vi "Set Relay State.vi"(8 "error in (no error)":errorcluster, 9 "relay action (Close Relay)":T1=enum."Close Relay", 10 "SLSC Switch in":refnum<class "SLSC Switch.lvclass">, 11 "PhysicalChannelRelay in":refnum<class "PhysicalChannelRelay.lvclass">) -> (0 "error out":errorcluster, 2 "SLSC Switch out":refnum<class "SLSC Switch.lvclass">, 3 "PhysicalChannelRelay out":refnum<class "PhysicalChannelRelay.lvclass">)   [LabVIEW 2015, in "PhysicalChannelRelay.lvclass"]
uses:
  PhysicalChannelRelay.lvclass
  slscsl/RelayAction.ctl
  SLSC Switch/SLSC Switch.lvclass
  SLSC Switch/SLSC Switch.lvclass/SLSC Switch.ctl
  PhysicalChannelRelay.lvclass/PhysicalChannelRelay.ctl
  <vilib>/SLSC/Set Phys Chan Property (Bool).vi
  <vilib>/SLSC/Commit Properties for Phys Chans.vi
  slscsl/slscsl.lvclass
  <vilib>/SLSC/SLSC.lvlib
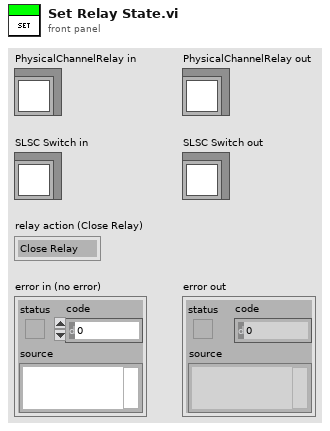
[diagram p1: front panel]
types:
  T1 = typedef "slscsl.lvclass/RelayAction.ctl" = enum16{"Open Relay", "Close Relay"}
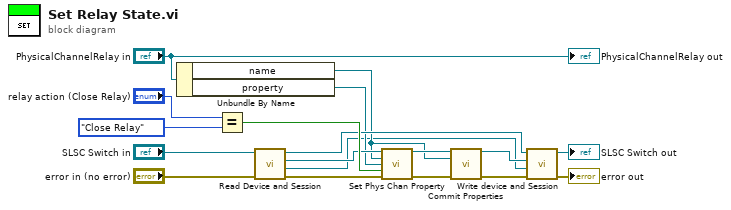
[diagram p0: block diagram]
diagram:
  n1 = Unbundle By Name("PhysicalChannelRelay in") -> ("name"=w2:refnum<k21>, "property"=w8:refnum<k21>)
  n2 = Equal?(x="relay action (Close Relay)", y=RelayAction."Close Relay") -> (x = y?=w17:bool)
  n3 = call "Read Device and Session.vi"("error in (no error)"="error in (no error)", "SLSC Switch in"="SLSC Switch in") -> ("error out"=w5:errorcluster, "device"=w1:refnum<k21>, "session"=w10:refnum<k21>, "SLSC Switch out"=w12:refnum<class "SLSC Switch.lvclass">)  [unwired: 6 in]
  n4 = call-poly <vilib>:"Set Phys Chan Property.vi"("session in"=w10, "physical channels"=w2, "property"=w8, "property value"=w17, "error in (no error)"=w5) -> ("session out"=w16:refnum<k21>, "error out"=w15:errorcluster)  [unwired: 9 in]
  n5 = call-poly <vilib>:"Commit Properties.vi"("session in"=w16, "physical channels"=w2, "error in (no error)"=w15) -> ("session out"=w9:refnum<k21>, "error out"=w4:errorcluster)  [unwired: 11 in]
  n6 = call "Write device and Session.vi"("error in (no error)"=w4, "device"=w1, "session"=w9, "SLSC Switch in"=w12) -> ("error out"=→"error out":errorcluster, "SLSC Switch out"=→"SLSC Switch out":refnum<class "SLSC Switch.lvclass">)  [unwired: 6 in]
  "PhysicalChannelRelay out" <- "PhysicalChannelRelay in"
